vi "handler_404.vi"(8 "error in (no error)":errorcluster, 11 "HTTP Request in":T1) -> (0 "error out":errorcluster, 3 "HTTP Request out":T1)   [LabVIEW 2011]
uses:
  http_request_response.ctl
  http_request.ctl
  http_field.ctl
  http_response.ctl
  template_field.ctl
  template_field_type.ctl
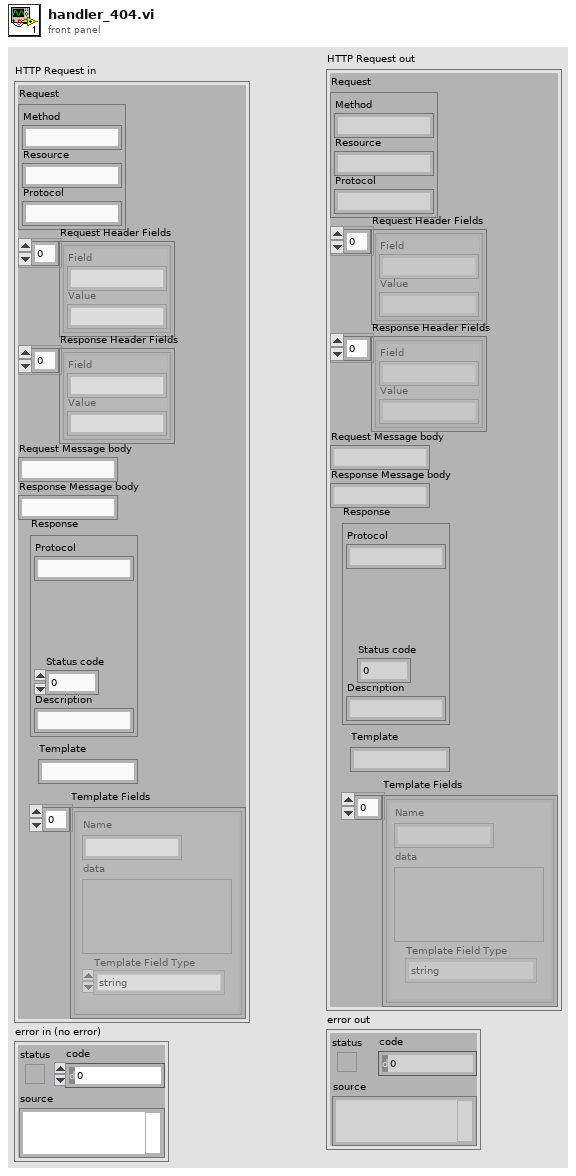
[diagram p1: front panel]
types:
  T1 = typedef "http_request_response.ctl" = cluster{"Request":T2, "Request Header Fields":T3[], "Response Header Fields":T3[], "Request Message body":string, "Response Message body":string, "Response":T4, "Template":string, "Template Fields":T5[]}
  T2 = typedef "http_request.ctl" = cluster{"Method":string, "Resource":string, "Protocol":string}
  T3 = typedef "http_field.ctl" = cluster{"Field":string, "Value":string}
  T4 = typedef "http_response.ctl" = cluster{"Protocol":string, "Status code":dbl, "Description":string}
  T5 = typedef "template_field.ctl" = cluster{"Name":string, "Template Field Type":T6, "data":variant}
  T6 = typedef "template_field_type.ctl" = enum16{"string", "string array", "number", "number array", "cluster", "cluster array"}
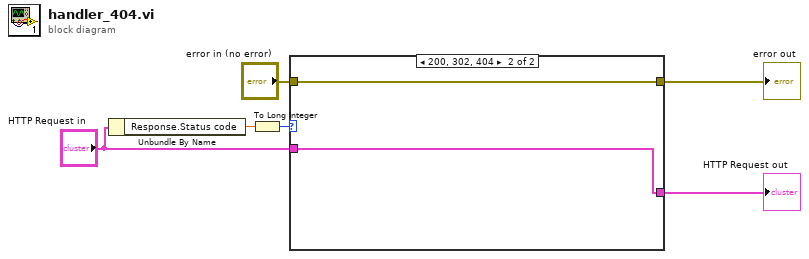
[diagram p0: block diagram]
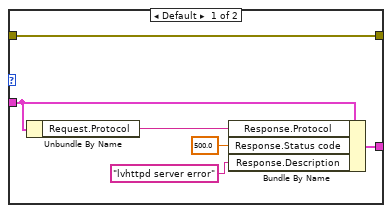
[diagram p2: hidden frame]
diagram:
  n1 = Unbundle By Name("HTTP Request in") -> ("Response.Status code"=w2:dbl)
  n2 = To Long Integer(number=w2) -> (32bit integer=w1:i32)
  n3 = case shown="200, 302, 404" w1 {
    tunnel: "HTTP Request in" -> [w10 w14]
    tunnel: [w11 w14] -> w5
    tunnel: "error in (no error)" -> [w12 w13]
    tunnel: [w12 w13] -> w4
    frame Default {
      n4 = Unbundle By Name(w10) -> ("Request.Protocol"=w9:string)
      n5 = Bundle By Name(cluster=w10, "Response.Protocol"=w9, "Response.Status code"=500.0, "Response.Description"="lvhttpd server error") -> (w11:T1)
    }
    frame 200, 302, 404 {
    }
  }
  "HTTP Request out" <- w5
  "error out" <- w4
